vi "Bimanual Target.vi"() -> ()   [LabVIEW 2013]
uses:
  Common/classes/PXI/PXI.lvclass
  Common/controls/Task Definition.ctl
  Common/controls/Task Types.ctl
  Common/classes/GripsMaster/GripsMaster.lvclass
  Common/labview_msgs/sensor_msgs/JointState.ctl
  Common/controls/Analog Values.ctl
panel:
  out "left_joint_angles":dbl[](array[numeric])
  out "UDP Receiver Status":errorcluster
  out "UDP Sender Status":errorcluster
  in  "ROS Machine":T1
  out "right_joint_angles":dbl[](array[numeric])
  in  "Stop":bool
  out "Labview Status":errorcluster
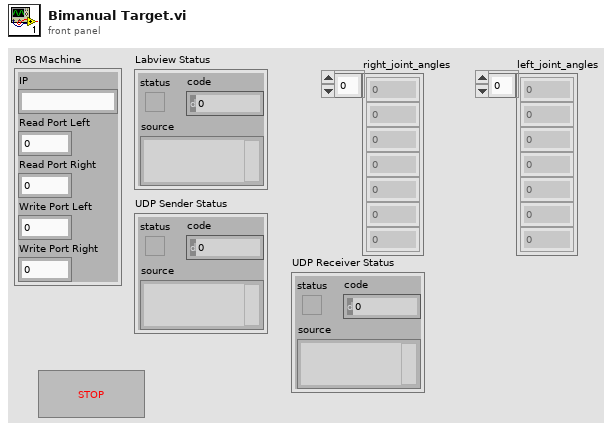
[diagram p1: front panel]
types:
  T1 = cluster{"IP":string, "Read Port Left":u16, "Read Port Right":u16, "Write Port Left":u16, "Write Port Right":u16}
  T2 = typedef "Task Definition.ctl" = cluster{"task_type":T3, "names":string[], "physical channels":tag, "min_value":dbl, "max_value":dbl, "task_number":i32}
  T3 = typedef "Task Types.ctl" = enum16{"Analog Input", "Analog Output", "Digital Input", "Digital Output"}
  T4 = enum16{"big-endian, network order", "native, host order", "little-endian"}
  T5 = typedef "JointState.ctl" = cluster{"header":cluster{"seq":u32, "stamp":cluster{"sec":i32, "nsec":i32}, "frame_id":string}, "name":string[], "position":dbl[], "velocity":dbl[], "effort":dbl[]}
  T6 = typedef "Digital Values.ctl" = cluster{"names":string[], "values":bool[]}
  T7 = typedef "Analog Values.ctl" = cluster{"names":string[], "values":dbl[]}
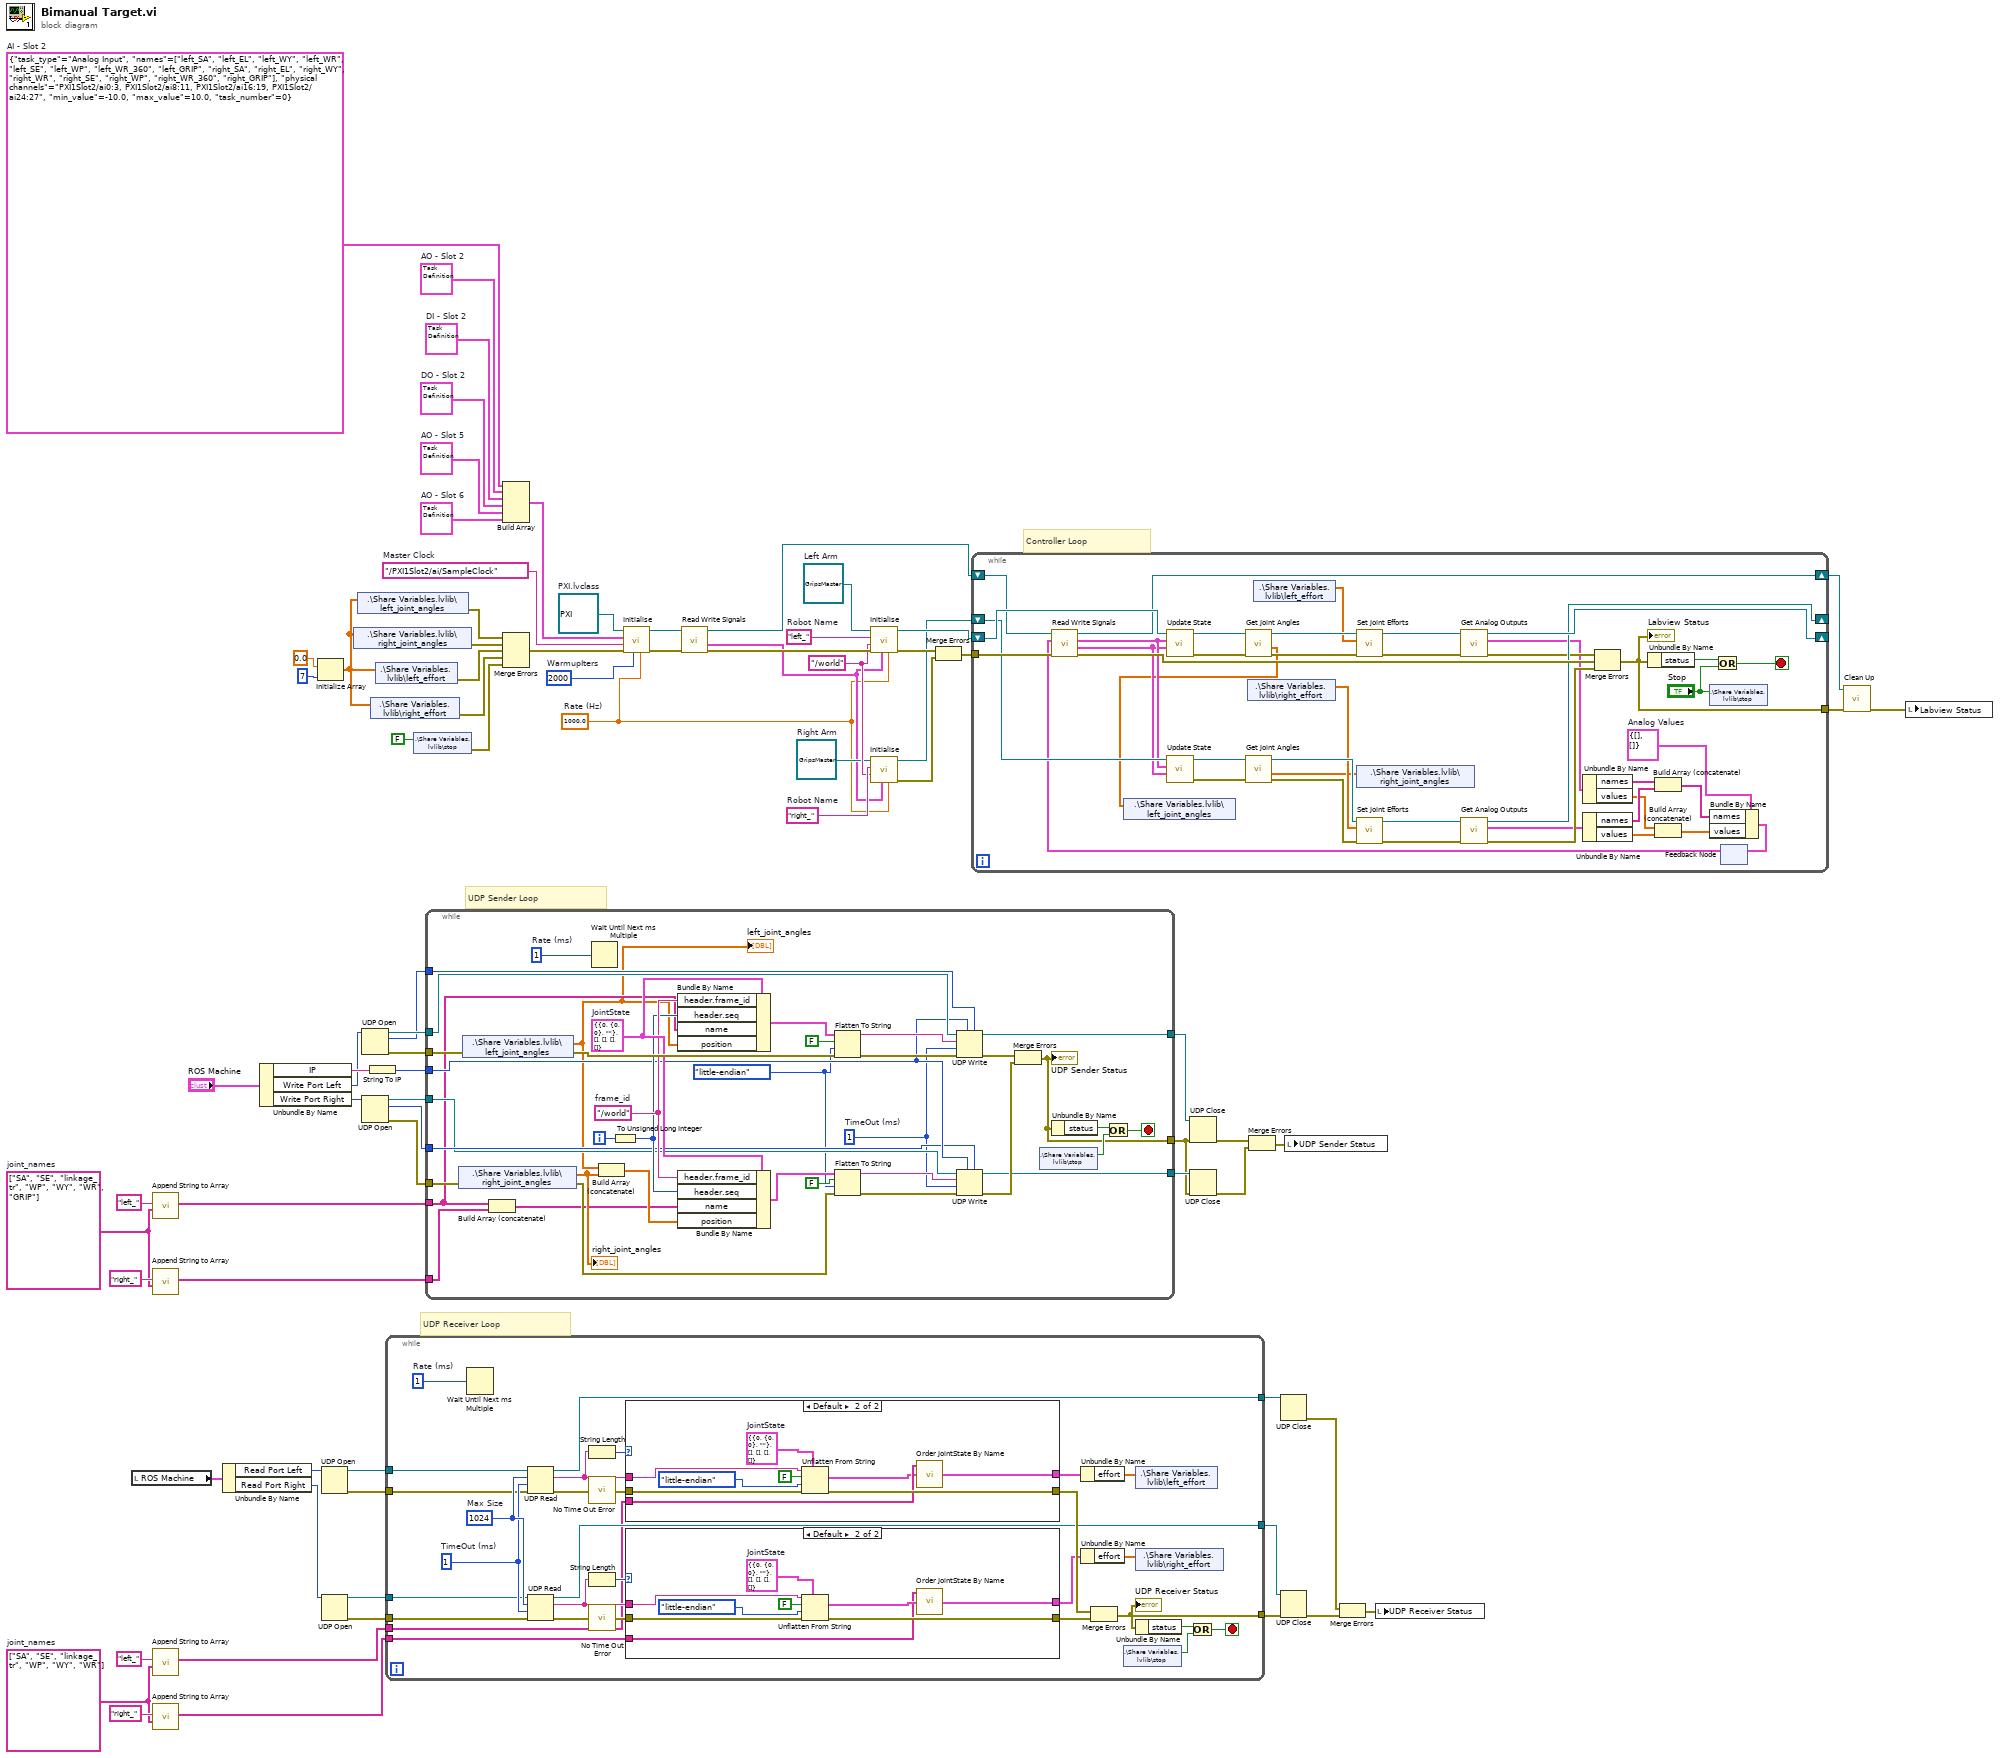
[diagram p0: block diagram]
diagram:
  w5 = string[] ["SA", "SE", "linkage_tr", "WP", "WY", "WR"]  # joint_names
  w43 = string[] ["SA", "SE", "linkage_tr", "WP", "WY", "WR", "GRIP"]  # joint_names
  w56 = "right_"  # Robot Name
  w50 = refnum<class "GripsMaster.lvclass"> refnum  # Right Arm
  w55 = "/world" ("Robot Frame")
  w66 = "left_"  # Robot Name
  w67 = refnum<class "GripsMaster.lvclass"> refnum  # Left Arm
  w1 = 1000.0  # Rate (Hz)
  w70 = u32 2000  # WarmupIters
  w71 = T2 {"task_type"=enum."Analog Output", "names"=["right_WY_FIX", "right_WY_CTR", "right_WP_FIX", "right_WP_CTR", "right_EL_FIX", "right_EL_CTR", "right_SA_FIX", "right_SA_CTR"], "physical channels"="PXI1Slot6/ao0:7", "min_value"=-2.0, "max_value"=2.0, "task_number"=0}  # AO - Slot 6
  w76 = T2 {"task_type"=enum."Analog Output", "names"=["left_WY_FIX", "left_WY_CTR", "left_WP_FIX", "left_WP_CTR", "left_EL_FIX", "left_EL_CTR", "left_SA_FIX", "left_SA_CTR"], "physical channels"="PXI1Slot5/ao0:7", "min_value"=-2.0, "max_value"=2.0, "task_number"=0}  # AO - Slot 5
  w74 = T2 {"task_type"=enum."Analog Output", "names"=["left_SE_FIX", "left_SE_CTR", "right_SE_FIX", "right_SE_CTR"], "physical channels"="PXI1Slot2/ao0:3", "min_value"=-2.0, "max_value"=2.0, "task_number"=0}  # AO - Slot 2
  w72 = T2 {"task_type"=enum."Digital Output", "names"=["left_halt", "left_wrist", "left_hyd", "left_gripper", "right_halt", "right_wrist", "right_hyd", "right_gripper"], "physical channels"="PXI1Slot2/port0/line4:7, PXI1Slot2/port0/line12:15", "min_value"=0.0, "max_value"=0.0, "task_number"=0}  # DO - Slot 2
  w73 = T2 {"task_type"=enum."Digital Input", "names"=["left_gripper", "left_wrist", "left_halt", "left_hyd", "right_gripper", "right_wrist", "right_halt", "right_hyd"], "physical channels"="PXI1Slot2/port0/line0:3, PXI1Slot2/port0/line8:11", "min_value"=0.0, "max_value"=0.0, "task_number"=0}  # DI - Slot 2
  w77 = T2 {"task_type"=enum."Analog Input", "names"=["left_SA", "left_EL", "left_WY", "left_WR", "left_SE", "left_WP", "left_WR_360", "left_GRIP", "right_SA", "right_EL", "right_WY", "right_WR", "right_SE", "right_WP", "right_WR_360", "right_GRIP"], "physical channels"="PXI1Slot2/ai0:3, PXI1Slot2/ai8:11, PXI1Slot2/ai16:19, PXI1Slot2/ai24:27", "min_value"=-10.0, "max_value"=10.0, "task_number"=0}  # AI - Slot 2
  w78 = tag "/PXI1Slot2/ai/SampleClock"  # Master Clock
  w79 = refnum<class "PXI.lvclass"> refnum  # PXI.lvclass
  # "UDP Receiver Loop"
  # "UDP Sender Loop"
  # "Controller Loop"
  n1 = local read "ROS Machine"() -> (w32:T1)
  n2 = call "Append String to Array.vi"("array"=w43, "name"="left_") -> ("result"=w47:string[])  [unwired: 9 in]
  n3 = call "Append String to Array.vi"("array"=w43, "name"="right_") -> ("result"=w42:string[])  [unwired: 9 in]
  n4 = call "Append String to Array.vi"("array"=w5, "name"="left_") -> ("result"=w3:string[])  [unwired: 9 in]
  n5 = call "Append String to Array.vi"("array"=w5, "name"="right_") -> ("result"=w4:string[])  [unwired: 9 in]
  n6 = Unbundle By Name(w32) -> ("Read Port Left"=w31:u16, "Read Port Right"=w30:u16)
  n7 = Unbundle By Name("ROS Machine") -> ("IP"=w45:string, "Write Port Left"=w36:u16, "Write Port Right"=w35:u16)
  n8 = Initialize Array(0.0 ("element"), 7 ("dimension size")) -> (w8:dbl[])
  n9 = UDP Open(11:w31) -> (port=w29:refnum<k16>, 0:w25:errorcluster)  [unwired: 1 in, 4 out]
  n10 = UDP Open(11:w30) -> (port=w28:refnum<k16>, 0:w24:errorcluster)  [unwired: 1 in, 4 out]
  n11 = shared-variable ".\\Share Variables.lvlib\\right_joint_angles"(w8) -> (error out=w13:errorcluster)  [unwired: 1 in]
  n12 = shared-variable ".\\Share Variables.lvlib\\left_joint_angles"(w8) -> (error out=w14:errorcluster)  [unwired: 1 in]
  n13 = UDP Open(11:w36) -> (port=w60:refnum<k16>, 0:w26:errorcluster, 2:w59:u16)  [unwired: 1 in, 3 out]
  n14 = UDP Open(11:w35) -> (port=w34:refnum<k16>, 0:w27:errorcluster, 2:w37:u16)  [unwired: 1 in, 3 out]
  n15 = String To IP(1:w45) -> (0:w58:u32)
  n16 = shared-variable ".\\Share Variables.lvlib\\right_effort"(w8) -> (error out=w11:errorcluster)  [unwired: 1 in]
  n17 = shared-variable ".\\Share Variables.lvlib\\left_effort"(w8) -> (error out=w12:errorcluster)  [unwired: 1 in]
  n18 = while {
    tunnel: w29 -> [w101]
    tunnel: w28 -> [w100]
    tunnel: w25 -> [w99]
    tunnel: w24 -> [w98]
    tunnel: [w89] -> w23
    tunnel: [w88] -> w19
    tunnel: [w86] -> w22
    tunnel: w4 -> [w81]
    tunnel: w3 -> [w80]
    stop <- w107 stop-if-true
    w102 = u32 1  # Rate (ms)
    w104 = 1024  # Max Size
    w103 = 1  # TimeOut (ms)
    n19 = Wait Until Next ms Multiple(millisecond multiple=w102) -> ()  [unwired: 1 out]
    n20 = UDP Read(connection ID=w101, max size (548)=w104, timeout ms (25000)=w103, 8:w99) -> (data out=w94:string, error out=w106:errorcluster, 3:w89:refnum<k16>)  [unwired: 2 out]
    n21 = UDP Read(connection ID=w100, max size (548)=w104, timeout ms (25000)=w103, 8:w98) -> (data out=w90:string, error out=w105:errorcluster, 3:w86:refnum<k16>)  [unwired: 2 out]
    n22 = String Length(string=w94) -> (length=w97:i32)
    n23 = call <vilib>:"No Time Out Error.vi"("error in (no error)"=w106) -> ("error out"=w96:errorcluster)  [unwired: 14 out]
    n24 = String Length(string=w90) -> (length=w91:i32)
    n25 = call <vilib>:"No Time Out Error.vi"("error in (no error)"=w105) -> ("error out"=w93:errorcluster)  [unwired: 14 out]
    n26 = case shown="Default" w97 {
      tunnel: [w119 w125] -> w95
      tunnel: w96 -> [w119 w126]
      tunnel: w94 -> [_ w123]
      tunnel: [_ w121] -> w85
      tunnel: w80 -> [_ w122]
      frame 0 {
      }
      frame Default {
        w124 = T5 {"header"={"seq"=0, "stamp"={"sec"=0, "nsec"=0}, "frame_id"=""}, "name"=[], "position"=[], "velocity"=[], "effort"=[]}  # JointState
        n27 = Unflatten From String(type=w124, binary string=w123, data includes array or string size? (T)=FALSE, byte order (0:big-endian, network order)=T4."little-endian", error in (no error)=w126) -> (value=w120:T5, error out=w125:errorcluster)  [unwired: 1 out]
        n28 = call "Order JointState By Name.vi"("Ordered Joint Names"=w122, "JointState In"=w120) -> ("JointState Out"=w121:T5)  [unwired: 7 in]
      }
    }
    n29 = case shown="Default" w91 {
      tunnel: [w109 w115] -> w92
      tunnel: w93 -> [w109 w116]
      tunnel: [_ w111] -> w82
      tunnel: w90 -> [_ w113]
      tunnel: w81 -> [_ w110]
      frame 0 {
      }
      frame Default {
        w114 = T5 {"header"={"seq"=0, "stamp"={"sec"=0, "nsec"=0}, "frame_id"=""}, "name"=[], "position"=[], "velocity"=[], "effort"=[]}  # JointState
        n30 = Unflatten From String(type=w114, binary string=w113, data includes array or string size? (T)=FALSE, byte order (0:big-endian, network order)=T4."little-endian", error in (no error)=w116) -> (value=w112:T5, error out=w115:errorcluster)  [unwired: 1 out]
        n31 = call "Order JointState By Name.vi"("Ordered Joint Names"=w110, "JointState In"=w112) -> ("JointState Out"=w111:T5)  [unwired: 7 in]
      }
    }
    n32 = Unbundle By Name(w85) -> ("effort"=w84:dbl[])
    n33 = Unbundle By Name(w82) -> ("effort"=w83:dbl[])
    n34 = Merge Errors(w95, w92) -> (w88:errorcluster)
    "UDP Receiver Status" <- w88
    n35 = shared-variable ".\\Share Variables.lvlib\\stop"() -> (w108:bool)  [unwired: 1 in, 1 out]
    n36 = shared-variable ".\\Share Variables.lvlib\\left_effort"(w84) -> ()  [unwired: 1 in, 1 out]
    n37 = shared-variable ".\\Share Variables.lvlib\\right_effort"(w83) -> ()  [unwired: 1 in, 1 out]
    n38 = Unbundle By Name(w88) -> ("status"=w87:bool)
    n39 = Or(x=w87, y=w108) -> (x .or. y?=w107:bool)
  }
  n40 = shared-variable ".\\Share Variables.lvlib\\stop"(FALSE ("stop")) -> (error out=w10:errorcluster)  [unwired: 1 in]
  n41 = while {
    tunnel: [w161] -> w61
    tunnel: w60 -> [w160]
    tunnel: w59 -> [w159]
    tunnel: w47 -> [w131]
    tunnel: w58 -> [w140]
    tunnel: w42 -> [w132]
    tunnel: [w141] -> w38
    tunnel: w37 -> [w139]
    tunnel: w34 -> [w138]
    tunnel: w26 -> [w153]
    tunnel: [w142] -> w33
    tunnel: w27 -> [w135]
    i -> [w162]
    stop <- w157 stop-if-true
    w136 = T4."little-endian" ("Byte order")
    w152 = T5 {"header"={"seq"=0, "stamp"={"sec"=0, "nsec"=0}, "frame_id"=""}, "name"=[], "position"=[], "velocity"=[], "effort"=[]}  # JointState
    w151 = "/world"  # frame_id
    w156 = u32 1  # Rate (ms)
    w137 = 1  # TimeOut (ms)
    n42 = shared-variable ".\\Share Variables.lvlib\\right_joint_angles"(error in=w135) -> (w134:dbl[], error out=w147:errorcluster)
    "right_joint_angles" <- w134
    n43 = shared-variable ".\\Share Variables.lvlib\\left_joint_angles"(error in=w153) -> (w129:dbl[], error out=w154:errorcluster)
    "left_joint_angles" <- w129
    n44 = Build Array (concatenate)(w131, w132) -> (w130:string[])
    n45 = Wait Until Next ms Multiple(millisecond multiple=w156) -> ()  [unwired: 1 out]
    n46 = Build Array (concatenate)(w129, w134) -> (w133:dbl[])
    n47 = To Unsigned Long Integer(number=w162) -> (unsigned 32bit integer=w150:u32)
    n48 = Bundle By Name(cluster=w152, "header.frame_id"=w151, "header.seq"=w150, "name"=w131, "position"=w129) -> (w163:T5)
    n49 = Bundle By Name(cluster=w152, "header.frame_id"=w151, "header.seq"=w150, "name"=w130, "position"=w133) -> (w148:T5)
    n50 = Flatten To String(anything=w163, prepend array or string size? (T)=FALSE, byte order (0:big-endian, network order)=w136, error in (no error)=w154) -> (data string=w165:string, error out=w164:errorcluster)  [unwired: 1 out]
    n51 = Flatten To String(anything=w148, prepend array or string size? (T)=FALSE, byte order (0:big-endian, network order)=w136, error in (no error)=w147) -> (data string=w146:string, error out=w145:errorcluster)  [unwired: 1 out]
    n52 = UDP Write(address=w140, port or service name=w159, connection ID=w160, data in=w165, 8:w164, 9:w137) -> (error out=w144:errorcluster, 3:w161:refnum<k16>)
    n53 = UDP Write(address=w140, port or service name=w139, connection ID=w138, data in=w146, 8:w145, 9:w137) -> (error out=w143:errorcluster, 3:w141:refnum<k16>)
    n54 = Merge Errors(w144, w143) -> (w142:errorcluster)
    "UDP Sender Status" <- w142
    n55 = shared-variable ".\\Share Variables.lvlib\\stop"() -> (w155:bool)  [unwired: 1 in, 1 out]
    n56 = Unbundle By Name(w142) -> ("status"=w158:bool)
    n57 = Or(x=w158, y=w155) -> (x .or. y?=w157:bool)
  }
  n58 = Build Array(w77, w74, w73, w72, w76, w71) -> (w75:T2[])
  n59 = Merge Errors(w14, w13, w12, w11, w10) -> (w9:errorcluster)
  n60 = call "Initialise.vi"("Rate (Hz)"=w1, "WarmupIters"=w70, "error in (no error)"=w9, "Master Clock"=w78, "Tasks Info"=w75, "PXI in"=w79) -> ("error out"=w68:errorcluster, "PXI out"=w69:refnum<class "PXI.lvclass">)  [unwired: 4 in]
  n61 = call "Read Write Signals.vi"("error in (no error)"=w68, "PXI in"=w69) -> ("error out"=w57:errorcluster, "Digital Inputs"=w2:T6, "PXI out"=w65:refnum<class "PXI.lvclass">)  [unwired: 6 in, 1 out]
  n62 = call "Initialise.vi"("Rate (Hz)"=w1, "Initial DI"=w2, "error in (no error)"=w57, "Robot Frame"=w55, "Robot Name"=w66, "Master in"=w67) -> ("error out"=w54:errorcluster, "Master out"=w62:refnum<class "GripsMaster.lvclass">)  [unwired: 4 in]
  n63 = call "Initialise.vi"("Rate (Hz)"=w1, "Initial DI"=w2, "Robot Frame"=w55, "Robot Name"=w56, "Master in"=w50) -> ("error out"=w53:errorcluster, "Master out"=w51:refnum<class "GripsMaster.lvclass">)  [unwired: 5 in]
  n64 = Merge Errors(w54, w53) -> (w52:errorcluster)
  n65 = while {
    tunnel: w52 -> [w205]
    tunnel: [w201] -> w63
    shift-right: [w204] -> w64
    shift-left: w65 -> [w206]
    shift-right: [w190] -> _
    shift-left: w62 -> [w209]
    shift-right: [w187] -> _
    shift-left: w51 -> [w199]
    stop <- w203 stop-if-true
    w178 = T7 {"names"=[], "values"=[]}  # Analog Values
    n66 = shared-variable ".\\Share Variables.lvlib\\right_effort"() -> (w169:dbl[])  [unwired: 1 in, 1 out]
    n67 = shared-variable ".\\Share Variables.lvlib\\left_effort"() -> (w183:dbl[])  [unwired: 1 in, 1 out]
    n68 = shared-variable ".\\Share Variables.lvlib\\stop"("Stop") -> ()  [unwired: 1 in, 1 out]
    n69 = feedback #1() -> (w170:T7)  [unwired: 1 in]
    n70 = call "Read Write Signals.vi"("error in (no error)"=w205, "Analog Outputs"=w170, "PXI in"=w206) -> ("error out"=w198:errorcluster, "Digital Inputs"=w194:T6, "Analog Inputs"=w195:T7, "PXI out"=w204:refnum<class "PXI.lvclass">)  [unwired: 5 in]
    n71 = call "Update State.vi"("Digital Inputs"=w194, "Analog Inputs"=w195, "GripsMaster in"=w209) -> ("error out"=w207:errorcluster, "GripsMaster out"=w208:refnum<class "GripsMaster.lvclass">)  [unwired: 7 in]
    n72 = call "Update State.vi"("Digital Inputs"=w194, "Analog Inputs"=w195, "GripsMaster in"=w199) -> ("error out"=w197:errorcluster, "GripsMaster out"=w196:refnum<class "GripsMaster.lvclass">)  [unwired: 7 in]
    n73 = call "Get Joint Angles.vi"("error in (no error)"=w207, "GripsMaster in"=w208) -> ("error out"=w185:errorcluster, "simulator_angles"=w167:dbl[], "GripsMaster out"=w191:refnum<class "GripsMaster.lvclass">)  [unwired: 6 in, 1 out]
    n74 = shared-variable ".\\Share Variables.lvlib\\left_joint_angles"(w167) -> ()  [unwired: 1 in, 1 out]
    n75 = call "Get Joint Angles.vi"("error in (no error)"=w197, "GripsMaster in"=w196) -> ("error out"=w186:errorcluster, "simulator_angles"=w168:dbl[], "GripsMaster out"=w182:refnum<class "GripsMaster.lvclass">)  [unwired: 6 in, 1 out]
    n76 = call "Set Joint Efforts.vi"("error in (no error)"=w185, "joint_efforts"=w183, "GripsMaster in"=w191) -> ("error out"=w192:errorcluster, "GripsMaster out"=w193:refnum<class "GripsMaster.lvclass">)  [unwired: 7 in]
    n77 = shared-variable ".\\Share Variables.lvlib\\right_joint_angles"(w168) -> ()  [unwired: 1 in, 1 out]
    n78 = call "Set Joint Efforts.vi"("error in (no error)"=w186, "joint_efforts"=w169, "GripsMaster in"=w182) -> ("error out"=w188:errorcluster, "GripsMaster out"=w189:refnum<class "GripsMaster.lvclass">)  [unwired: 7 in]
    n79 = call "Get Analog Outputs.vi"("error in (no error)"=w192, "GripsMaster in"=w193) -> ("error out"=w181:errorcluster, "Analog Values"=w180:T7, "GripsMaster out"=w190:refnum<class "GripsMaster.lvclass">)  [unwired: 7 in]
    n80 = call "Get Analog Outputs.vi"("error in (no error)"=w188, "GripsMaster in"=w189) -> ("error out"=w184:errorcluster, "Analog Values"=w179:T7, "GripsMaster out"=w187:refnum<class "GripsMaster.lvclass">)  [unwired: 7 in]
    n81 = Unbundle By Name(w180) -> ("names"=w177:string[], "values"=w174:dbl[])
    n82 = Unbundle By Name(w179) -> ("names"=w176:string[], "values"=w173:dbl[])
    n83 = Merge Errors(w181, w198, w184) -> (w201:errorcluster)
    "Labview Status" <- w201
    n84 = Unbundle By Name(w201) -> ("status"=w202:bool)
    n85 = Build Array (concatenate)(w177, w176) -> (w175:string[])
    n86 = Build Array (concatenate)(w174, w173) -> (w172:dbl[])
    n87 = Bundle By Name(cluster=w178, "names"=w175, "values"=w172) -> (w171:T7)
    n88 = Or(x=w202, y="Stop") -> (x .or. y?=w203:bool)
    n89 = feedback-in #1(w171) -> ()
  }
  n90 = UDP Close(connection ID=w61, 8:w33) -> (error out=w41:errorcluster)  [unwired: 1 out]
  n91 = UDP Close(connection ID=w38, 8:w33) -> (error out=w40:errorcluster)  [unwired: 1 out]
  n92 = Merge Errors(w41, w40) -> (w39:errorcluster)
  n93 = UDP Close(connection ID=w23) -> (error out=w18:errorcluster)  [unwired: 1 in, 1 out]
  n94 = UDP Close(connection ID=w22, 8:w19) -> (error out=w20:errorcluster)  [unwired: 1 out]
  n95 = local write "UDP Sender Status"(w39) -> ()
  n96 = Merge Errors(w18, w20) -> (w21:errorcluster)
  n97 = local write "UDP Receiver Status"(w21) -> ()
  n98 = call "Clean Up.vi"("error in (no error)"=w63, "PXI in"=w64) -> ("error out"=w49:errorcluster)  [unwired: 8 in, 1 out]
  n99 = local write "Labview Status"(w49) -> ()
